vi "Read.vi"   [LabVIEW 2017, in "ADCMT 6240.lvlib"]
doc: "This VI read one or more measurements from the instrument."
uses:
  ADCMT 6240.lvlib
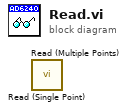
[diagram p0: block diagram]
diagram:
  n1 = call "Read (Single Point).vi"() -> ()  [unwired: 9 in, 7 out]
  n2 = call "Read (Multiple Points).vi"() -> ()  [unwired: 9 in, 7 out]
